vi "Configure IIC Trigger Source.vi"(0 "VISA resource name":refnum<visa-resource-name>, 1 "Type (0: Start Condition)":u16(ring) items=["Start Condition", "Stop Condition", "Missing Acknowledge", "Restart", "EEPROM Data Read", "Frame(Start:Addr7:Read:Ack:Data)", "Frame(Start:Addr7:Write:Ack:Data)", "10 - bit Write"], 3 "EEPROM Qualifier (1: Not Equal)":u16(ring)=1 items=["Equal", "Not Equal", "Less Than", "Greater Than"], 5 "Serial Clock Source (0: Channel 1)":u16(ring) items=["Channel 1", "Channel 2", "Channel 3", "Channel 4", "DIG 0", "DIG 1", "DIG 2", "DIG 3", "DIG 4", "DIG 5", "DIG 6", "DIG 7", "DIG 8", "DIG 9", "DIG 10", "DIG 11", "DIG 12", "DIG 13", "DIG 14", "DIG 15", "EXT"], 9 "Serial Data Source (1: Channel 2)":u16(ring)=1 items=["Channel 1", "Channel 2", "Channel 3", "Channel 4", "DIG 0", "DIG 1", "DIG 2", "DIG 3", "DIG 4", "DIG 5", "DIG 6", "DIG 7", "DIG 8", "DIG 9", "DIG 10", "DIG 11", "DIG 12", "DIG 13", "DIG 14", "DIG 15", "EXT"], 11 "error in (no error)":errorcluster, 12 "Address (-1)":i32=-1, 14 "Data (-1)":i32=-1) -> (4 "VISA resource name out":refnum<visa-resource-name>, 15 "error out":errorcluster)   [LabVIEW 2017, in "Agilent 6000 Series.lvlib"]
doc: "This VI configures the IIC trigger. You specify the clock source with the Serial Clock Source parameter, data source with the Serial Data Source parameter and type with the Type parameter and the IIC data with the Address and Data parameters.\n\n<B>NOTE:</B>\n\nThis VI is only valid for 6000 Series models. An error will be thrown if this VI is run with 5000 Series scopes."
uses:
  <instrlib>/Agilent 6000 Series/Agilent 6000 Series.lvlib
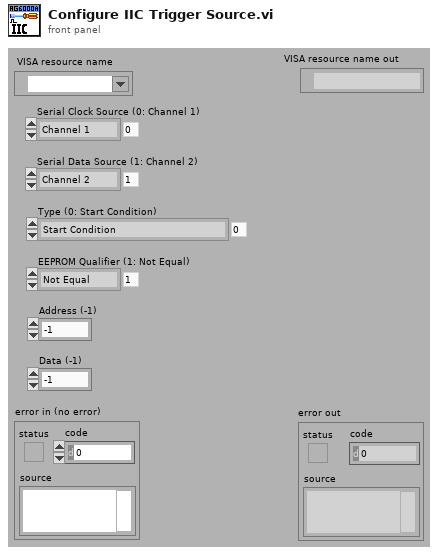
[diagram p1: front panel]
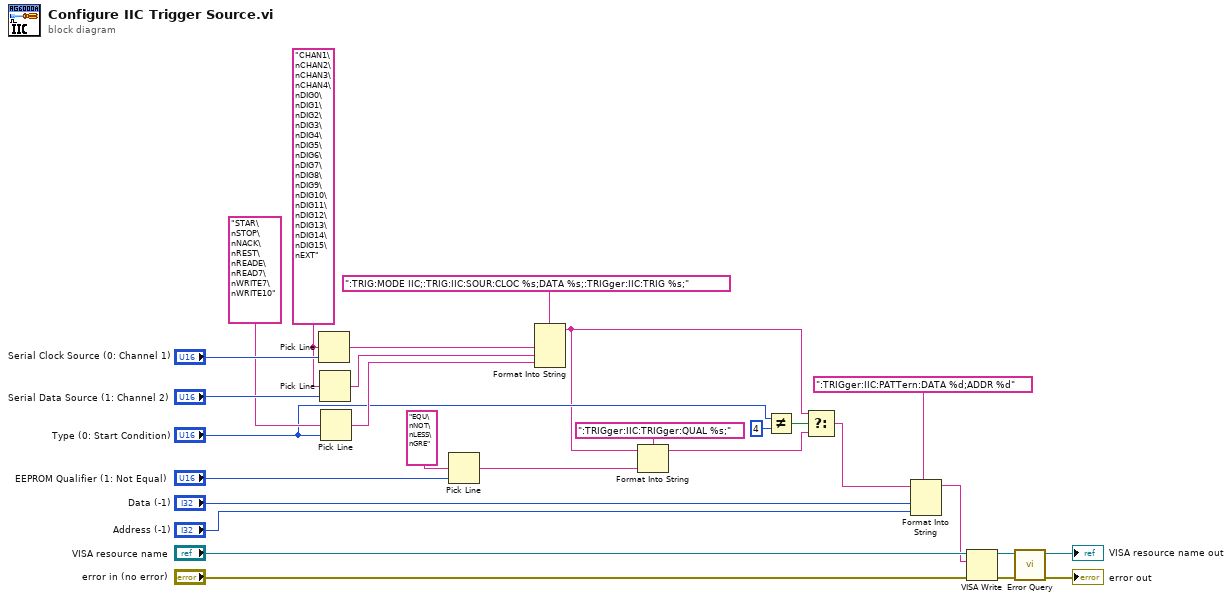
[diagram p0: block diagram]
diagram:
  w19 = "CHAN1\nCHAN2\nCHAN3\nCHAN4\nDIG0\nDIG1\nDIG2\nDIG3\nDIG4\nDIG5\nDIG6\nDIG7\nDIG8\nDIG9\nDIG10\nDIG11\nDIG12\nDIG13\nDIG14\nDIG15\nEXT"
  n1 = Pick Line(multi-line string=w19, line index="Serial Clock Source (0: Channel 1)") -> (output string=w20:string)  [unwired: 1 in]
  n2 = Pick Line(multi-line string=w19, line index="Serial Data Source (1: Channel 2)") -> (output string=w17:string)  [unwired: 1 in]
  n3 = Pick Line(multi-line string="STAR\nSTOP\nNACK\nREST\nREADE\nREAD7\nWRITE7\nWRITE10", line index="Type (0: Start Condition)") -> (output string=w15:string)  [unwired: 1 in]
  n4 = Pick Line(multi-line string="EQU\nNOT\nLESS\nGRE", line index="EEPROM Qualifier (1: Not Equal)") -> (output string=w10:string)  [unwired: 1 in]
  n5 = Format Into String(format string=":TRIG:MODE IIC;:TRIG:IIC:SOUR:CLOC %s;DATA %s;:TRIGger:IIC:TRIG %s;" ("Source Command"), w20, w17, w15) -> (resulting string=w8:string)  [unwired: 2 in, 1 out]
  n6 = Format Into String(format string=":TRIGger:IIC:TRIGger:QUAL %s;", initial string=w8, w10) -> (resulting string=w7:string)  [unwired: 1 in, 1 out]
  n7 = Not Equal?(x="Type (0: Start Condition)", y=u16 4) -> (x != y?=w11:bool)
  n8 = Select(t=w8, s=w11, f=w7) -> (s? t:f=w2:string)
  n9 = Format Into String(format string=":TRIGger:IIC:PATTern:DATA %d;ADDR %d", initial string=w2, "Data (-1)", "Address (-1)") -> (resulting string=w1:string)  [unwired: 1 in, 1 out]
  n10 = VISA Write(VISA resource name="VISA resource name", write buffer=w1, error in (no error)="error in (no error)") -> (VISA resource name out=w24:refnum<visa-resource-name>, error out=w23:errorcluster)  [unwired: 1 out]
  n11 = call <instrlib>:"Error Query.vi"("error in (no error)"=w23, "VISA resource name"=w24) -> ("error out"=→"error out":errorcluster, "VISA resource name out"=→"VISA resource name out":refnum<visa-resource-name>)  [unwired: 6 in, 2 out]
